vi "motors.vi"   [LabVIEW 2013]
uses:
  <vilib>/myRIO/Instrument Drivers/Onboard IO/DIO/vis/Smart Open.vi
  <vilib>/myRIO/Instrument Drivers/Onboard IO/DIO/vis/Write.vi
  <vilib>/myRIO/Instrument Drivers/Onboard IO/PWM/vis/Smart Open.vi
  <vilib>/myRIO/Instrument Drivers/Onboard IO/PWM/vis/Set Duty Cycle and Frequency.vi
  <vilib>/myRIO/Instrument Drivers/Onboard IO/DIO/vis/Open.vi
  <vilib>/myRIO/Instrument Drivers/Onboard IO/PWM/vis/Open.vi
  <vilib>/myRIO/Common/Instrument Driver Framework/myRIO v1.0/DIO/vis/myRIO v1.1 Open DIO.vi
  <vilib>/myRIO/Common/Instrument Driver Framework/myRIO v1.0/PWM/vis/myRIO v1.1 Open PWM.vi
  <vilib>/myRIO/Common/Instrument Driver Framework/Utilities/vis/Validate Channels.vi
  <vilib>/myRIO/Common/Instrument Driver Framework/myRIO v1.0/DIO/vis/myRIO v1.0 Reserve DIO.vi
  <vilib>/myRIO/Common/Instrument Driver Framework/myRIO v1.0/PWM/vis/myRIO v1.0 Reserve PWM.vi
  <vilib>/myRIO/Common/Instrument Driver Framework/myRIO v1.0/Resource Manager/vis/myRIO v1.0 Reserve Channel List.vi
  <vilib>/myRIO/Common/Instrument Driver Framework/myRIO v1.0/DIO/vis/myRIO v1.0 Build MUX Configuration DIO.vi
  <vilib>/myRIO/Common/Instrument Driver Framework/myRIO v1.0/PWM/vis/myRIO v1.0 Build MUX Configuration PWM.vi
  <vilib>/myRIO/Common/Instrument Driver Framework/myRIO v1.0/Resource Manager/vis/myRIO v1.0 Reserve Channel.vi
  <vilib>/myRIO/Common/Instrument Driver Framework/myRIO v1.0/Resource Manager/vis/myRIO v1.0 Unreserve Channel.vi
  <vilib>/myRIO/Common/Instrument Driver Framework/myRIO v1.0/Resource Manager/vis/myRIO v1.0 Create Configuration List.vi
  <vilib>/myRIO/Common/Instrument Driver Framework/myRIO v1.0/Resource Manager/vis/myRIO v1.0 Build Mutex Name.vi
  <vilib>/myRIO/Common/Instrument Driver Framework/myRIO v1.0/myRIO v1.1 Open.vi
  <vilib>/Utility/VariantDataType/GetNumericInfo.vi
  <vilib>/Utility/error.llb/Error Cluster From Error Code.vi
  <vilib>/myRIO/Common/Instrument Driver Framework/Utilities/vis/IO Manager.vi
  <vilib>/myRIO/Common/Instrument Driver Framework/Utilities/vis/Configuration Manager.vi
  <vilib>/myRIO/Common/Instrument Driver Framework/myRIO v1.0/Resource Manager/vis/myRIO v1.0 Configure IO.vi
  <vilib>/myRIO/Common/Instrument Driver Framework/myRIO v1.0/myRIO v1.0 Close.vi
  <vilib>/myRIO/Common/Instrument Driver Framework/myRIO v1.0/DIO/vis/myRIO v1.0 Write DIO.vi
  <vilib>/myRIO/Common/Instrument Driver Framework/myRIO v1.0/PWM/vis/myRIO v1.0 Write PWM.vi
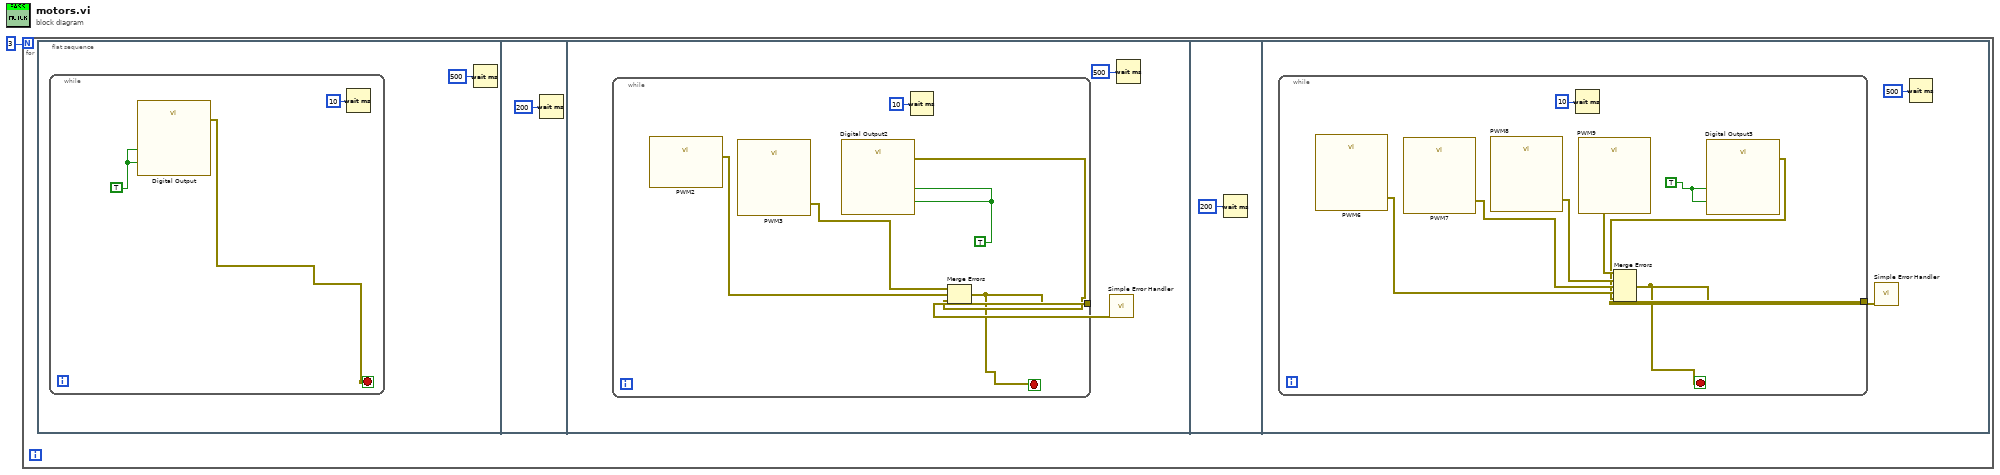
[diagram p0: block diagram]
diagram:
  n1 = for {
    N: 3 -> [_]
    n2 = flat-sequence {
      frame #0 {
        n3 = while {
          stop <- w3 stop-if-true
          w4 = TRUE
          n4 = call "Digital Output"("DIR (A/DIO1 (Pin 13))"=w4, "PWM (A/DIO0 (Pin 11))"=w4) -> ("error out"=w3:errorcluster)  [unwired: 25 in]
          n5 = Wait (ms)(milliseconds to wait=u32 10) -> ()  [unwired: 1 out]
        }
        n6 = Wait (ms)(milliseconds to wait=u32 500) -> ()  [unwired: 1 out]
      }
      frame #1 {
        n7 = Wait (ms)(milliseconds to wait=u32 200) -> ()  [unwired: 1 out]
      }
      frame #2 {
        n8 = while {
          tunnel: [w9] -> w7
          stop <- w9 stop-if-true
          w10 = TRUE
          n9 = call "PWM2"() -> ("error out"=w13:errorcluster)  [unwired: 27 in]
          n10 = call "PWM3"() -> ("error out"=w12:errorcluster)  [unwired: 27 in]
          n11 = call "Digital Output2"("A/DIO2 (Pin 15)"=w10, "A/DIO3 (Pin 17)"=w10) -> ("error out"=w11:errorcluster)  [unwired: 25 in]
          n12 = Wait (ms)(milliseconds to wait=u32 10) -> ()  [unwired: 1 out]
          n13 = Merge Errors(w12, w13, w11) -> (w9:errorcluster)
        }
        n14 = call <vilib>:"Simple Error Handler.vi"("error in (no error)"=w7) -> ()  [unwired: 4 in, 5 out]
        n15 = Wait (ms)(milliseconds to wait=u32 500) -> ()  [unwired: 1 out]
      }
      frame #3 {
        n16 = Wait (ms)(milliseconds to wait=u32 200) -> ()  [unwired: 1 out]
      }
      frame #4 {
        n17 = while {
          tunnel: [w18] -> w17
          stop <- w18 stop-if-true
          w20 = TRUE
          n18 = call "PWM6"() -> ("error out"=w24:errorcluster)  [unwired: 27 in]
          n19 = call "PWM7"() -> ("error out"=w23:errorcluster)  [unwired: 27 in]
          n20 = call "PWM8"() -> ("error out"=w22:errorcluster)  [unwired: 27 in]
          n21 = Wait (ms)(milliseconds to wait=u32 10) -> ()  [unwired: 1 out]
          n22 = call "PWM9"() -> ("error out"=w21:errorcluster)  [unwired: 27 in]
          n23 = call "Digital Output3"("MOTOR 3 (A/DIO4 (Pin 19))"=w20, "MOTOR 4 (A/DIO5 (Pin 21))"=w20) -> ("error out"=w19:errorcluster)  [unwired: 25 in]
          n24 = Merge Errors(w21, w22, w23, w24, w19) -> (w18:errorcluster)
        }
        n25 = call <vilib>:"Simple Error Handler.vi"("error in (no error)"=w17) -> ()  [unwired: 4 in, 5 out]
        n26 = Wait (ms)(milliseconds to wait=u32 500) -> ()  [unwired: 1 out]
      }
    }
  }
